vi "Acquire.vi"(8 "error in (no error)":errorcluster, 10 "Msg in":T1, 11 "PXIDigitizer in":refnum<class "TapeMonitor.lvclass">) -> (0 "error out":errorcluster, 1 "new command":string, 2 "Msg out":T1, 3 "PXIDigitizer out":refnum<class "TapeMonitor.lvclass">)   [LabVIEW 2020, in "TapeMonitor.lvclass"]
uses:
  TapeMonitor.lvclass
  C:/GEECS/Developers Version/source/Device Drivers/BaseDriver/BaseDriver.lvclass
  BaseDriver/DriverMsg.ctl
  analysis_data_typdef.ctl
  <vilib>/vision/Image Controls.llb/IMAQ Image.ctl
  shared/OnOffTypeDef.ctl
  TapeMonitor.lvclass/TapeMonitor.ctl
  shared/CompressAndUpdate(Poly)/CompressAndUpdate(Numeric).vi
  shared/CompressAndUpdate(Poly)/CompressAndUpdate(IMAQ Image).vi
  shared/CompressAndUpdate(Poly)/CompressAndUpdate(Enum).vi
  BaseDriver/BaseDriver.lvclass
  <vilib>/vision/NI_Vision_Development_Module.lvlib
  <vilib>/Analysis/NI_AALBase.lvlib
panel:
  out "Particle Measurements (Pixels)":dbl[][](array[numeric]) format="%.2f"
  out "Centroid":cluster{"X Centroid":sgl, "Y Centroid":sgl} {"Y Centroid" format="%.2f"; "X Centroid" format="%.2f"}
  out "shotnumber":i32
  out "TapeOK":bool
  out "FitnessLimit":dbl
  out "Number of Particles":i32=4
  out "symmetry":dbl=0.8279313704277508
  out "AreaSymmetry":dbl=0.8170854732403674
  out "fitness":dbl=0.7483901847989424
  out "sqrt(x)":dbl=0.9039278031128191
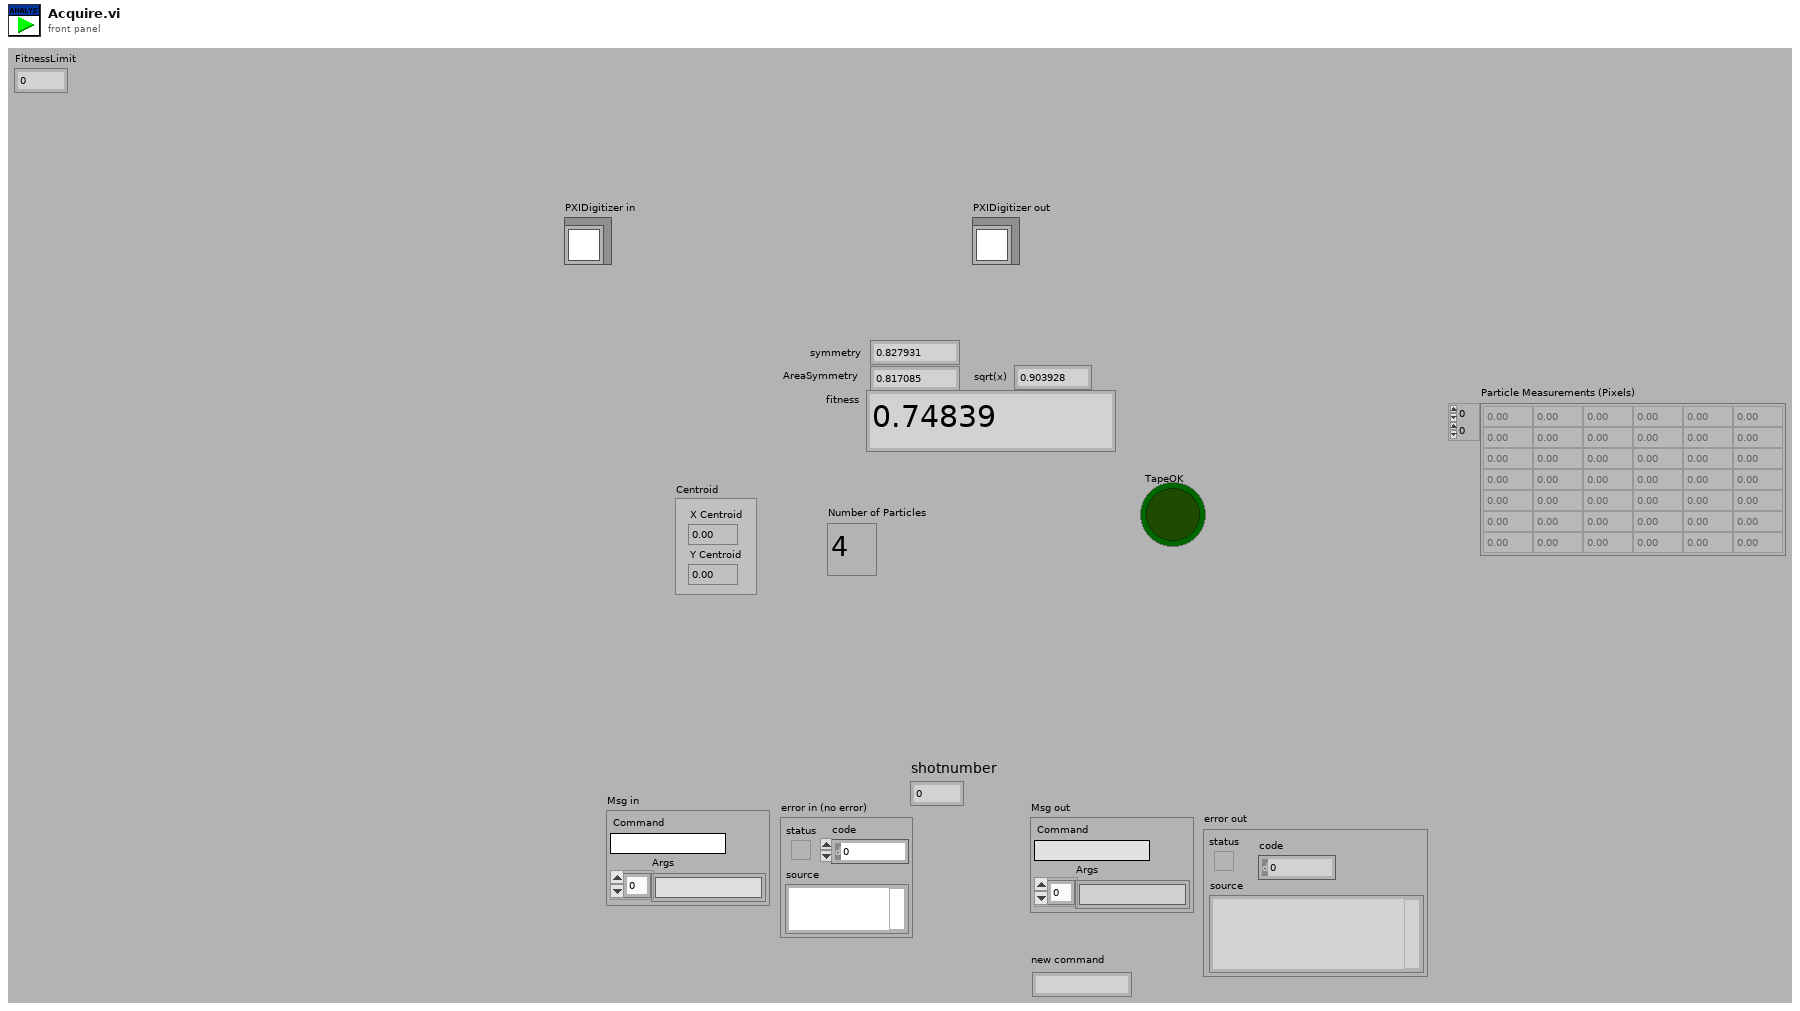
[diagram p1: front panel]
types:
  T1 = typedef "DriverMsg.ctl" = cluster{"Command":string, "Args":string[]}
  T2 = typedef "Particle Parameters" = i32
  T3 = cluster{"Measurement Parameter":T2, "Range Lower Value":dbl, "Range Upper Value":dbl, "Range":bool, "Measurement Type":bool}
  T4 = typedef "OnOffTypeDef.ctl" = enum16{"off", "on"}
  T5 = cluster{"Desired Font (Application)":enum16{"User-specified Font", "Application Font", "System Font", "Dialog Font"}, "[User-specified Font]":cluster{"Font Name":string, "Size":i16, "Strikeout?":bool, "Italic?":bool, "Underline?":bool, "Outline?":bool, "Shadow?":bool, "Bold?":bool, "Rotation Angle":dbl}, "Horizontal Alignment":i16, "Vertical Alignment":i16}
  T6 = cluster{"X Size":i32, "Y Size":i32, "Order #":i32}
  T7 = cluster{"Measurement Parameter":T2, "Range Lower Value":dbl, "Range Upper Value":dbl, "Range":bool, "Measurement Type":bool}[]
  T8 = typedef "Image Type" = u32
  T9 = typedef "TapeMonitor.lvclass/analysis_data_typdef.ctl" = cluster{"image":T10}
  T10 = typedef "IMAQ Image.ctl" = refnum<image>
  T11 = typedef "SubscriberCluster_TypDEf.ctl" = cluster{"tcp data event":T12, "Event Registration Refnum":refnum<event-registration>, "data queue":refnum<queue>, "Devices":string[], "Alias":string[], "Variable header":string[], "Devices ALL":string[]}
  T12 = typedef "tcp_new_data_event.ctl" = refnum<user-event>
  T13 = cluster{"Particle Measurements (Pixels)[0]":dbl, "Particle Measurements (Pixels)[1]":dbl, "Particle Measurements (Pixels)[2]":dbl, "Particle Measurements (Pixels)[3]":dbl}
  T14 = cluster{"Particle Measurements (Pixels)[0]":dbl, "Particle Measurements (Pixels)[1]":dbl}
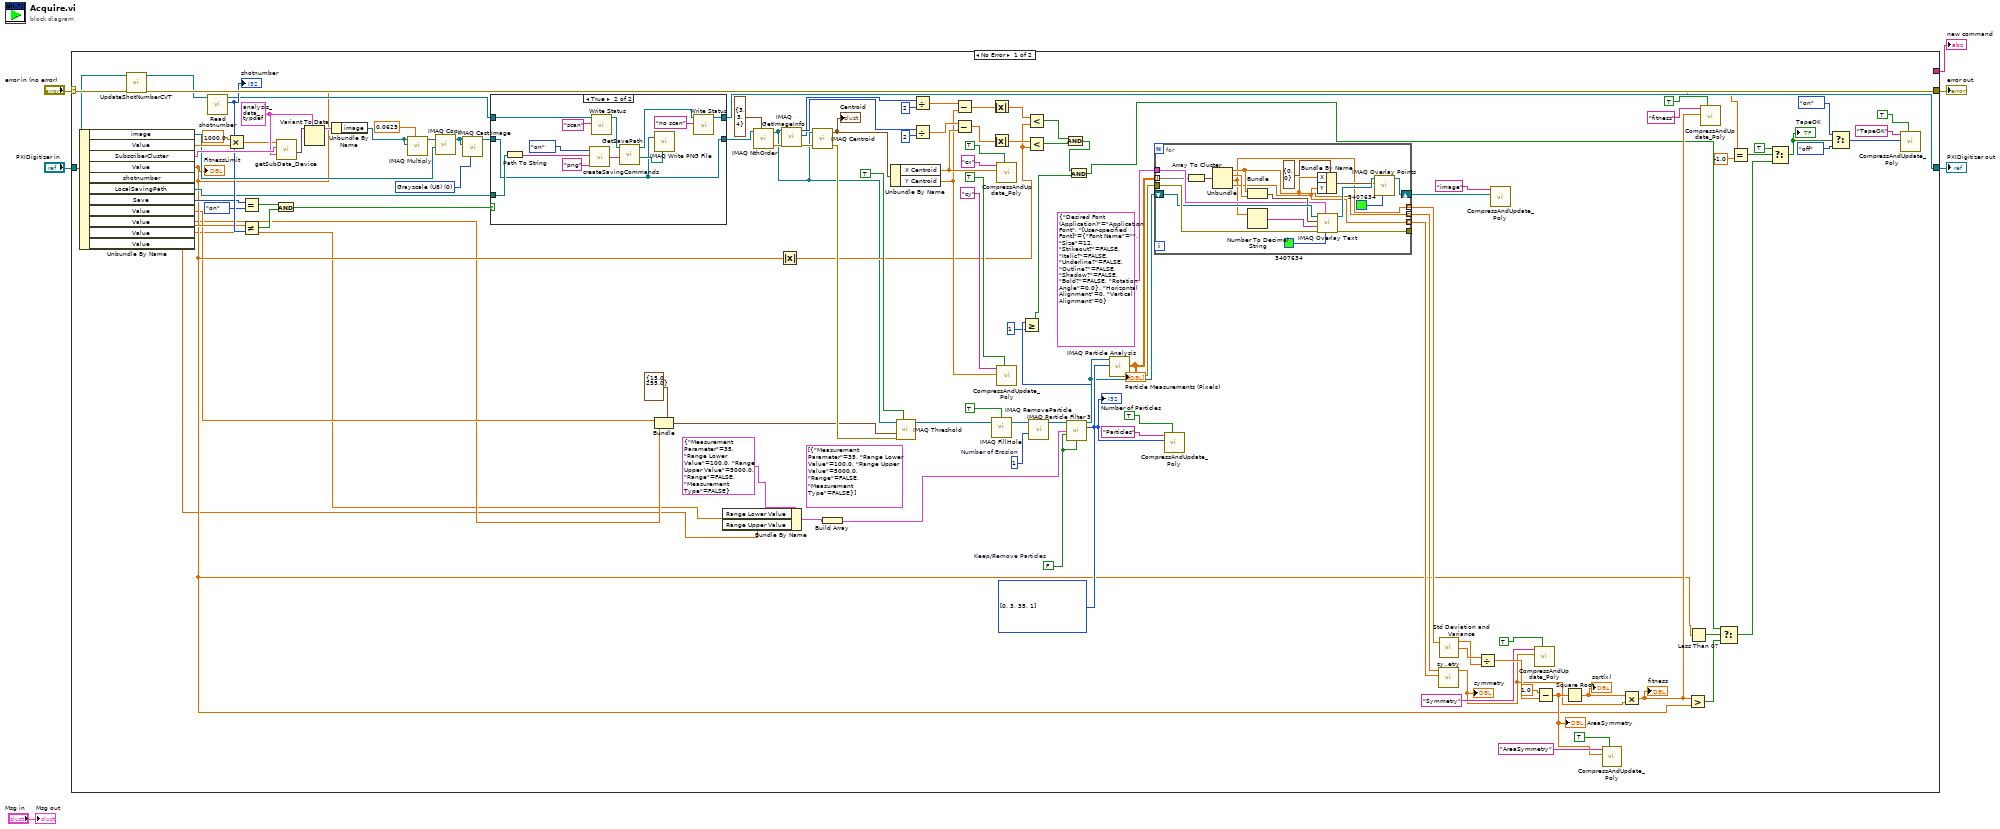
[diagram p0: block diagram]
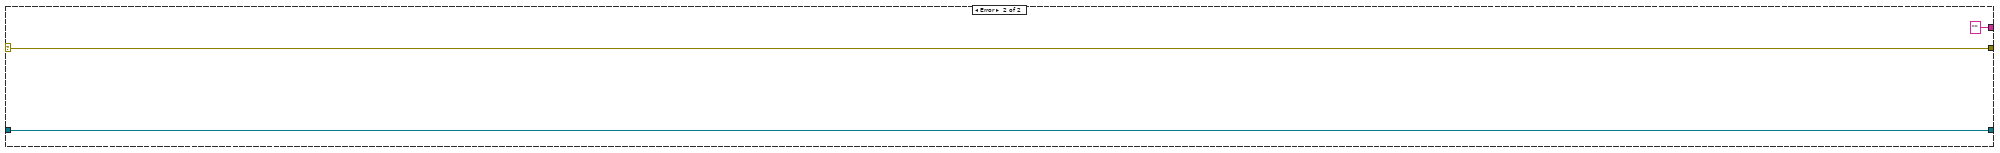
[diagram p3: hidden frame]
diagram:
  n1 = case shown="No Error" "error in (no error)" {
    selector: "error in (no error)" -> [w120 w155]
    tunnel: "PXIDigitizer in" -> [w70 w156]
    tunnel: [w66 w156] -> w6
    tunnel: [w113 w155] -> w4
    tunnel: [_ "" ("new command")] -> w1
    frame No Error {
      (unwired) T7 [{"Measurement Parameter"=35, "Range Lower Value"=100.0, "Range Upper Value"=5000.0, "Range"=FALSE, "Measurement Type"=FALSE}] ("Selection Values")
      w91 = T8 0 items=["Grayscale (U8)", "Grayscale (I16)", "Grayscale (SGL)", "Complex (CSG)", "RGB (U32)", "HSL (U32)", "RGB (U64)", "Grayscale (U16)"] ("Image Type")
      w103 = T2[] [0, 3, 35, 1] items=["Center of Mass X", "Center of Mass Y", "First Pixel X", "First Pixel Y", "Bounding Rect Left", "Bounding Rect Top", "Bounding Rect Right", "Bounding Rect Bottom", "Max Feret Diameter Start X", "Max Feret Diameter Start Y", "Max Feret Diameter End X", "Max Feret Diameter End Y", "Max Horiz. Segment Length Left", "Max Horiz. Segment Length Right", "Max Horiz. Segment Length Row", "-", "Bounding Rect Width", "Bounding Rect Height", "Bounding Rect Diagonal", "Perimeter", "Convex Hull Perimeter", "Holes' Perimeter", "Max Feret Diameter", "Equivalent Ellipse Major Axis", "Equivalent Ellipse Minor Axis", "Equivalent Ellipse Minor Axis (Feret)", "Equivalent Rect Long Side", "Equivalent Rect Short Side", "Equivalent Rect Diagonal", "Equivalent Rect Short Side (Feret)", "Average Horiz. Segment Length", "Average Vert. Segment Length", "Hydraulic Radius", "Waddel Disk Diameter", "-", "Area", "Holes' Area", "Particle & Holes' Area", "Convex Hull Area", "Image Area", "-", "Number of Holes", "Number of Horiz. Segments", "Number of Vert. Segments", "-", "Orientation", "Max Feret Diameter Orientation", "-", "% Area/Image Area", "% Area/(Particle & Holes' Area)", "Ratio of Equivalent Ellipse Axes", "Ratio of Equivalent Rect Sides", "-", "Elongation Factor", "Compactness Factor", "Heywood Circularity Factor", "Type Factor", "-", "Sum X", "Sum Y", "Sum XX", "Sum XY", "Sum YY", "Sum XXX", "Sum XXY", "Sum XYY", "Sum YYY", "-", "Moment of Inertia XX", "Moment of Inertia XY", "Moment of Inertia YY", "Moment of Inertia XXX", "Moment of Inertia XXY", "Moment of Inertia XYY", "Moment of Inertia YYY", "Norm. Moment of Inertia XX", "Norm. Moment of Inertia XY", "Norm. Moment of Inertia YY", "Norm. Moment of Inertia XXX", "Norm. Moment of Inertia XXY", "Norm. Moment of Inertia XYY", "Norm. Moment of Inertia YYY", "Hu Moment 1", "Hu Moment 2", "Hu Moment 3", "Hu Moment 4", "Hu Moment 5", "Hu Moment 6", "Hu Moment 7"] ("Pixel Measurements")
      w96 = FALSE  # Keep/Remove Particles
      w95 = 1  # Number of Erosion
      w117 = T9 {"image"=refnum} ("data")
      n2 = Unbundle By Name(w70) -> ("image"=w73:T10, "Value"=w116:dbl, "SubscriberCluster"=w119:T11, "Value"=w29:dbl, "shotnumber"=w69:dbl, "LocalSavingPath"=w67:path, "Save"=w64:T4, "Value"=w13:dbl, "Value"=w12:dbl, "Value"=w8:dbl, "Value"=w7:dbl)
      "FitnessLimit" <- w29
      n3 = call "UpdateShotNumberCVT.vi"("error in (no error)"=w120, "BaseDriver in"=w70) -> ("error out"=w113:errorcluster, "BaseDriver out"=w72:refnum<class "TapeMonitor.lvclass">)  [unwired: 8 in]
      n4 = call-dynamic "Read shotnumber.vi"("BaseDriver in"=w72) -> ("shotnumber"=w71:i32, "BaseDriver out"=w68:refnum<class "TapeMonitor.lvclass">)  [unwired: 7 in, 2 out]
      "shotnumber" <- w71
      n5 = Multiply(x=1000.0, y=w116) -> (x*y=w114:dbl)
      n6 = Equal?(x=w64, y=OnOffTypeDef."on" ("Settings.Save")) -> (x = y?=w62:bool)
      n7 = Not Equal?(x=w69, y=w71) -> (x != y?=w65:bool)
      n8 = And(x=w62, y=w65) -> (x .and. y?=w61:bool)
      n9 = call "getSubData_Device.vi"("variant in"=w117, "SubscriberCluster"=w119, "timeout"=w114) -> ("variant out"=w118:variant)  [unwired: 6 in, 2 out]
      n10 = Variant To Data(type=w117, Variant=w118) -> (data=w112:T9)  [unwired: 1 in, 1 out]
      n11 = Unbundle By Name(w112) -> ("image"=w18:T10)
      n12 = call "IMAQ Multiply"("Image Src A"=w18, "Constant"=sgl 0.0625, "Image Dst"=w18) -> ("Image Dst Out"=w59:T10)  [unwired: 4 in, 1 out]
      n13 = call "IMAQ Copy"("Image Dst"=w73, "Image Src"=w59) -> ("Image Dst Out"=w16:T10)  [unwired: 4 in, 1 out]
      n14 = call "IMAQ Cast Image"("Image Type"=w91, "Image Dst"=w16, "Image Src"=w16) -> ("Image Dst Out"=w17:T10)  [unwired: 7 in, 1 out]
      n15 = case shown="True" w61 {
        tunnel: w17 -> [w121 w123]
        tunnel: w68 -> [w122 w129]
        tunnel: w67 -> [_ w134]
        tunnel: [w122 w126] -> w66
        tunnel: [w121 w123] -> w20
        frame False {
        }
        frame True {
          n16 = Path To String(path=w134) -> (string=w132:string)
          n17 = call "createSavingCommands.vi"("extension"="png", "Saving Path (local)"=w132, "Save"=OnOffTypeDef."on") -> ("String"=w133:string)  [unwired: 1 in]
          n18 = call "Write Status.vi"("Status"="scan", "BaseDriver in"=w129) -> ("BaseDriver out"=w128:refnum<class "TapeMonitor.lvclass">)  [unwired: 8 in, 1 out]
          n19 = call-dynamic "GetSavePath.vi"("new command"=w133, "BaseDriver in"=w128) -> ("Path"=w135:path, "BaseDriver out"=w127:refnum<class "TapeMonitor.lvclass">)  [unwired: 5 in, 3 out]
          n20 = call "IMAQ Write PNG File"("File Path"=w135, "Image"=w123) -> ()  [unwired: 4 in, 3 out]
          n21 = call "Write Status.vi"("Status"="no scan", "BaseDriver in"=w127) -> ("BaseDriver out"=w126:refnum<class "TapeMonitor.lvclass">)  [unwired: 8 in, 1 out]
        }
      }
      n22 = Bundle(cluster=cluster{"Lower value":sgl, "Upper value":sgl} {"Lower value"=15.0, "Upper value"=255.0} ("Range 2"), "Lower value"=w13, "Upper value"=w12) -> (w14:cluster{"Lower value":sgl, "Upper value":sgl})
      n23 = Bundle By Name(cluster=T3 {"Measurement Parameter"=35, "Range Lower Value"=100.0, "Range Upper Value"=5000.0, "Range"=FALSE, "Measurement Type"=FALSE} ("Selection Value"), "Range Lower Value"=w8, "Range Upper Value"=w7) -> (w10:T3)
      n24 = call "IMAQ NthOrder"("Image Src"=w20, "Size & Order #"=T6 {"X Size"=3, "Y Size"=3, "Order #"=4} ("Size & Order # 2")) -> ("Image Dst Out"=w19:T10, "error out"=w37:errorcluster)  [unwired: 5 in]
      n25 = Absolute Value(x=w29) -> (abs(x)=w28:dbl)
      n26 = call "IMAQ GetImageInfo"("error in (no error)"=w37, "Image"=w19) -> ("error out"=w55:errorcluster, "Y Resolution"=w45:i32, "X Resolution"=w53:i32)  [unwired: 2 in, 5 out]
      n27 = call "IMAQ Centroid"("error in (no error)"=w55, "Image"=w19) -> ("error out"=w36:errorcluster, "Centroid"=w54:cluster{"X Centroid":sgl, "Y Centroid":sgl})  [unwired: 2 in]
      "Centroid" <- w54
      n28 = Build Array(w10) -> (w9:T7)
      n29 = Unbundle By Name(w54) -> ("X Centroid"=w35:sgl, "Y Centroid"=w34:sgl)
      n30 = call "IMAQ Threshold"("Keep/Replace Value (Replace)"=TRUE ("Keep/Replace Value (Replace) 2"), "error in (no error)"=w36, "Range"=w14, "Image Src"=w19) -> ("Image Dst Out"=w21:T10)  [unwired: 6 in, 1 out]
      n31 = Divide(x=w45, y=2) -> (x/y=w47:dbl)
      n32 = Divide(x=w53, y=2) -> (x/y=w51:dbl)
      n33 = Subtract(x=w47, y=w34) -> (x-y=w48:dbl)
      n34 = Subtract(x=w51, y=w35) -> (x-y=w50:dbl)
      n35 = Absolute Value(x=w48) -> (abs(x)=w44:dbl)
      n36 = Absolute Value(x=w50) -> (abs(x)=w49:dbl)
      n37 = call "IMAQ FillHole"("Image Src"=w21, "Connectivity 4/8 (8)"=TRUE) -> ("Image Dst Out"=w94:T10)  [unwired: 2 in, 3 out]
      n38 = call-poly "CompressAndUpdate_Poly.vi"("force CVT update (false)"=TRUE, "Numeric"=w35, "command or variable name"="cx") -> ()  [unwired: 8 in, 1 out]
      n39 = call-poly "CompressAndUpdate_Poly.vi"("force CVT update (false)"=TRUE, "Numeric"=w34, "command or variable name"="cy") -> ()  [unwired: 8 in, 1 out]
      n40 = Less?(x=w44, y=w28) -> (x < y?=w43:bool)
      n41 = Less?(x=w49, y=w28) -> (x < y?=w42:bool)
      n42 = call "IMAQ RemoveParticle"("Number of Erosion"=w95, "Image Src"=w94) -> ("Image Dst Out"=w97:T10)  [unwired: 5 in, 4 out]
      n43 = And(x=w43, y=w42) -> (x .and. y?=w27:bool)
      n44 = call "IMAQ Particle Filter 3"("Image Src"=w97, "Selection Values"=w9, "Keep/Remove Particles (F)"=w96, "Fill Holes? (F)"=w96) -> ("Image Dst Out"=w102:T10, "Number of Particles"=w26:i32)  [unwired: 5 in, 5 out]
      "Number of Particles" <- w26
      n45 = Greater Or Equal?(x=w26, y=1) -> (x >= y?=w24:bool)
      n46 = And(x=w27, y=w24) -> (x .and. y?=w23:bool)
      n47 = call "IMAQ Particle Analysis"("Pixel Measurements"=w103, "Image"=w102) -> ("error out"=w101:errorcluster, "Particle Measurements (Pixels)"=w99:dbl[][])  [unwired: 3 in, 5 out]
      "Particle Measurements (Pixels)" <- w99
      n48 = for {
        tunnel: w101 -> [w153]
        tunnel: [w152] -> _
        tunnel: T5 {"Desired Font (Application)"=enum."Application Font", "[User-specified Font]"={"Font Name"="", "Size"=12, "Strikeout?"=FALSE, "Italic?"=FALSE, "Underline?"=FALSE, "Outline?"=FALSE, "Shadow?"=FALSE, "Bold?"=FALSE, "Rotation Angle"=0.0}, "Horizontal Alignment"=0, "Vertical Alignment"=0} ("Font, Size & Style") -> [w145]
        tunnel: w99 -> [w144] mode=indexing
        tunnel: [w138] -> w105 mode=indexing
        tunnel: [w137] -> w104 mode=indexing
        tunnel: [w136] -> w106 mode=indexing
        shift-right: [w142] -> w22
        shift-left: w102 -> [w149]
        n49 = Array To Cluster(array=w144) -> (cluster=w148:T13)
        n50 = Unbundle(w148) -> ("Particle Measurements (Pixels)[0]"=w138:dbl, "Particle Measurements (Pixels)[1]"=w147:dbl, "Particle Measurements (Pixels)[2]"=w136:dbl, "Particle Measurements (Pixels)[3]"=w137:dbl)
        n51 = Bundle("Particle Measurements (Pixels)[0]"=w138, "Particle Measurements (Pixels)[1]"=w147) -> (w146:T14)  [unwired: 1 out]
        n52 = Number To Decimal String(number=w136) -> (decimal integer string=w151:string)  [unwired: 1 out]
        n53 = Bundle By Name(cluster=cluster{"X":i32, "Y":i32} {"X"=0, "Y"=0} ("Point"), "X"=w138, "Y"=w137) -> (w139:cluster{"X":i32, "Y":i32})
        n54 = call "IMAQ Overlay Text"("Text Color (black)"=u32 3407634, "Font, Size & Style"=w145, "error in (no error)"=w153, "String"=w151, "Origin"=w146, "Image"=w149) -> ("error out"=w152:errorcluster, "Image Out"=w143:T10)  [unwired: 2 in, 2 out]
        n55 = call "IMAQ Overlay Points"("Color"=u32 3407634 ("Text Color (black)"), "Point"=w139, "Image"=w143) -> ("Image Out"=w142:T10)  [unwired: 7 in, 1 out]
      }
      n56 = call-poly "CompressAndUpdate_Poly.vi"("force CVT update (false)"=TRUE, "Numeric"=w26, "command or variable name"="Particles") -> ()  [unwired: 8 in, 1 out]
      n57 = call "sy,,etry.vi"("Array 2"=w104, "Array"=w105) -> ("x-y 3"=w77:dbl)  [unwired: 9 in]
      "symmetry" <- w77
      n58 = call <vilib>:"Std Deviation and Variance.vi"("X"=w106) -> ("mean"=w107:dbl, "standard deviation"=w108:dbl)  [unwired: 1 in, 1 out]
      n59 = Divide(x=w108, y=w107) -> (x/y=w110:dbl)
      n60 = call-poly "CompressAndUpdate_Poly.vi"("IMAQ Image"=w22, "command or variable name"="image") -> ()  [unwired: 9 in, 1 out]
      n61 = call-poly "CompressAndUpdate_Poly.vi"("force CVT update (false)"=TRUE, "Numeric"=w77, "command or variable name"="Symmetry") -> ()  [unwired: 8 in, 1 out]
      n62 = Subtract(x=1.0 ("x/y"), y=w110) -> (x-y=w80:dbl)
      "AreaSymmetry" <- w80
      n63 = Square Root(x=w80) -> (sqrt(x)=w111:dbl)
      "sqrt(x)" <- w111
      n64 = call-poly "CompressAndUpdate_Poly.vi"("force CVT update (false)"=TRUE, "Numeric"=w80, "command or variable name"="AreaSymmetry") -> ()  [unwired: 8 in, 1 out]
      n65 = Multiply(x=w111, y=w77) -> (x*y=w84:dbl)
      "fitness" <- w84
      n66 = Greater?(x=w84, y=w29) -> (0:w40:bool)
      n67 = Less Than 0?(x=w29) -> (x < 0?=w41:bool)
      n68 = call-poly "CompressAndUpdate_Poly.vi"("force CVT update (false)"=TRUE, "Numeric"=w84, "command or variable name"="fitness") -> ()  [unwired: 8 in, 1 out]
      n69 = Select(t=w23, s=w41, f=w40) -> (s? t:f=w39:bool)
      n70 = Equal?(x=w29, y=-1.0) -> (x = y?=w57:bool)
      n71 = Select(t=TRUE, s=w57, f=w39) -> (s? t:f=w38:bool)
      "TapeOK" <- w38
      n72 = Select(t=OnOffTypeDef."on" ("Save"), s=w38, f=OnOffTypeDef."off" ("Save")) -> (s? t:f=w86:T4)
      n73 = call-poly "CompressAndUpdate_Poly.vi"("force CVT update (false)"=TRUE, "enum variant"=w86, "command or variable name"="TapeOK") -> ()  [unwired: 8 in, 1 out]
    }
    frame Error {
    }
  }
  "PXIDigitizer out" <- w6
  "error out" <- w4
  "new command" <- w1
  "Msg out" <- "Msg in"
